vi "Write Internal Message Queue.vi"(8 "error in (no error)":errorcluster, 10 "Internal Message Queue":refnum<queue>, 11 "Generic Controller in":refnum<class "Generic Plugin.lvclass">) -> (0 "error out":errorcluster, 3 "Generic Controller out":refnum<class "Generic Plugin.lvclass">)   [LabVIEW 2020, in "RxnRover.lvlib" / "Generic Plugin.lvclass"]
doc: "Assigns a message queue as the new Internal Message Queue used for internal communications in the Controller object."
uses:
  Generic Plugin.lvclass
  Sub VIs/Message Queue/Message Cluster.ctl
  Generic Plugin.lvclass/Generic Plugin.ctl
  Sub VIs/Message Queue/test Message Queue.lvlib
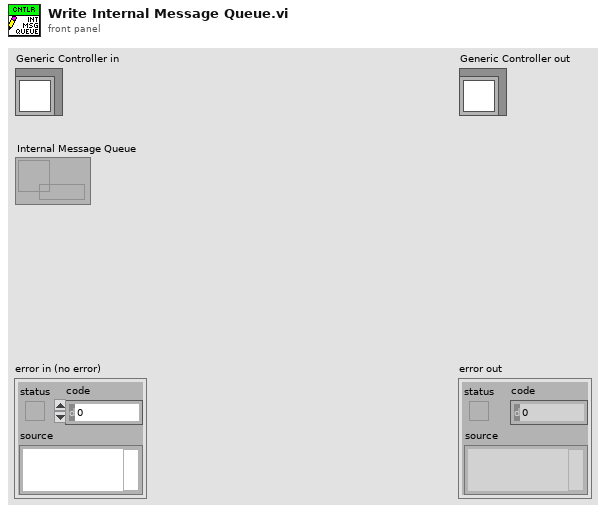
[diagram p1: front panel]
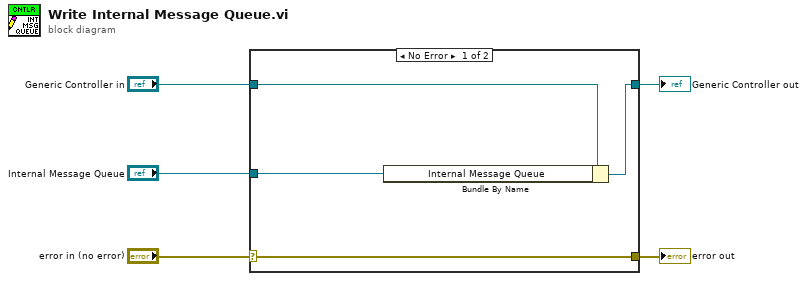
[diagram p0: block diagram]
diagram:
  n1 = case shown="No Error" "error in (no error)" {
    selector: "error in (no error)" -> [w9 w10]
    tunnel: [w9 w10] -> w4
    tunnel: [w7 w11] -> w2
    tunnel: "Generic Controller in" -> [w8 w11]
    tunnel: "Internal Message Queue" -> [w6 _]
    frame No Error {
      n2 = Bundle By Name(cluster=w8, "Internal Message Queue"=w6) -> (w7:refnum<class "Generic Plugin.lvclass">)
    }
    frame Error {
    }
  }
  "error out" <- w4
  "Generic Controller out" <- w2
